vi "Interpolate String.vi"(6 "Gantry in":refnum<class "Gantry.lvclass">, 8 "error in (no error)":errorcluster, 10 "Input String":string, 11 "gScript Interpreter in":refnum<class "gScript Interpreter.lvclass">) -> (0 "error out":errorcluster, 2 "Output String":string, 3 "gScript Interpreter out":refnum<class "gScript Interpreter.lvclass">, 4 "Gantry out":refnum<class "Gantry.lvclass">)   [LabVIEW 2026, in "gScript Interpreter.lvclass"]
uses:
  gScript Interpreter.lvclass
  Shared Components/Gantry Class/Gantry.lvclass
  <vilib>/regexp/Match Regular Expression.xnode
  gScript Interpreter.lvclass/gScript Interpreter.ctl
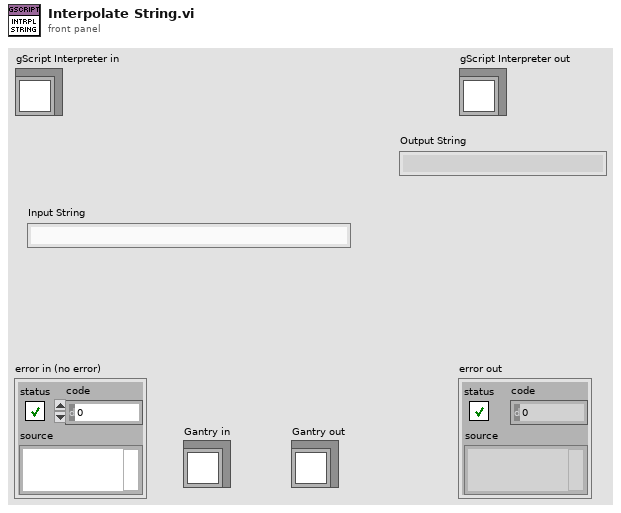
[diagram p1: front panel]
types:
  T1 = typedef "Memory Cell.ctl" = cluster{"type":T2, "x":dbl, "y":dbl, "z":dbl, "w":dbl}
  T2 = typedef "Memory Cell Type Enum.ctl" = enum16{"integer", "float", "vector", "rotation"}
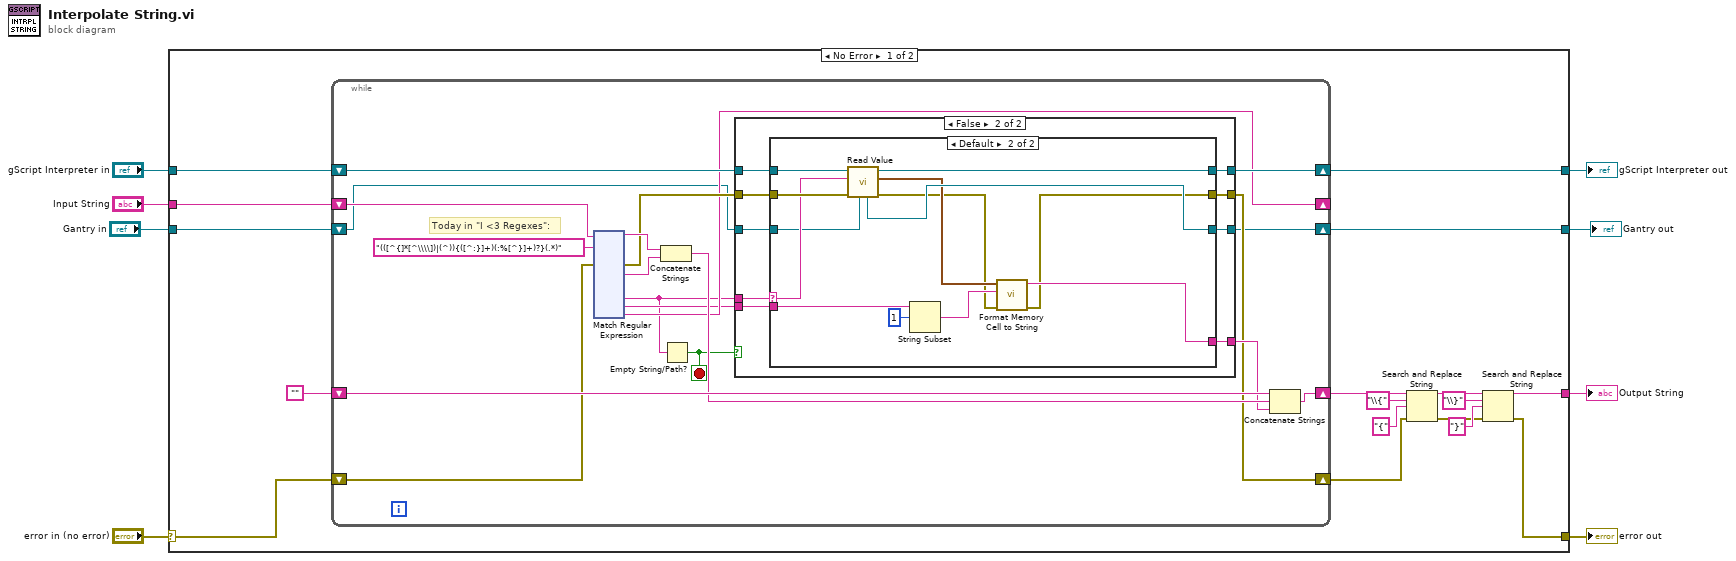
[diagram p0: block diagram]
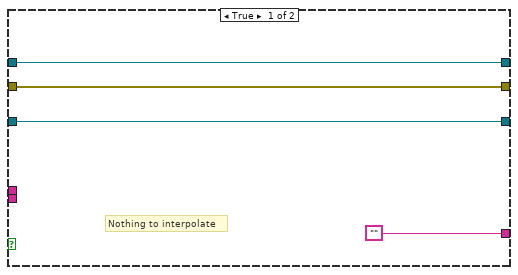
[diagram p2: hidden frame]
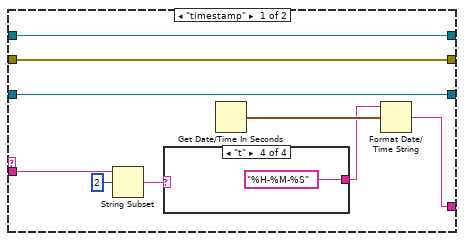
[diagram p3: hidden frame]
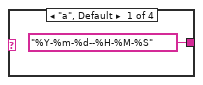
[diagram p4: hidden frame]
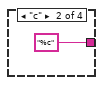
[diagram p5: hidden frame]
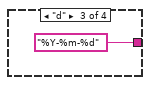
[diagram p6: hidden frame]
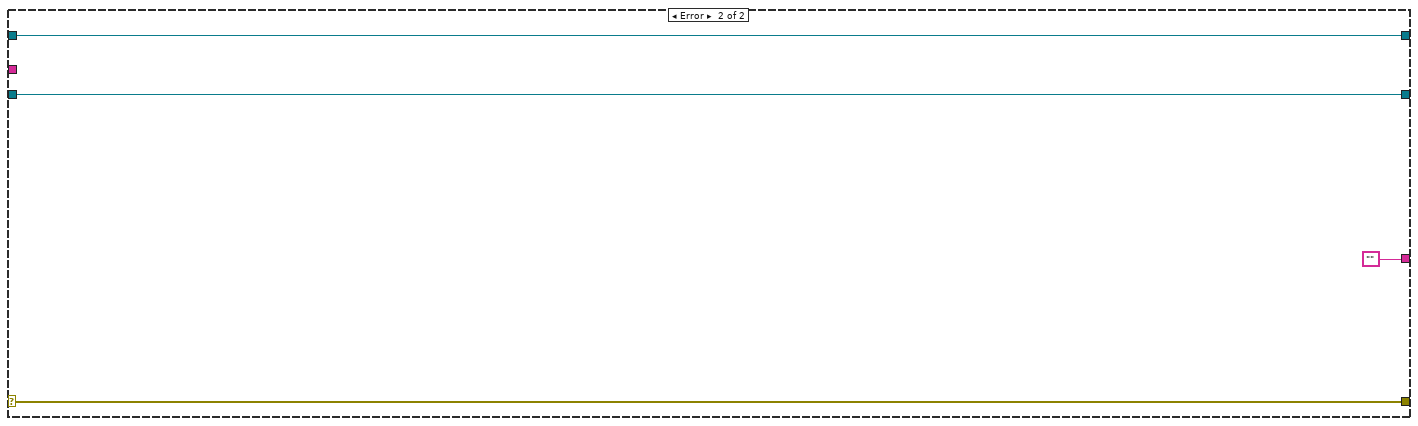
[diagram p7: hidden frame]
diagram:
  n1 = case shown="No Error" "error in (no error)" {
    selector: "error in (no error)" -> [w21 w211]
    tunnel: [w12 w211] -> w7
    tunnel: [w22 w210] -> w5
    tunnel: "gScript Interpreter in" -> [w23 w210]
    tunnel: "Input String" -> [w25 _]
    tunnel: [w11 ""] -> w3
    tunnel: "Gantry in" -> [w10 w208]
    tunnel: [w9 w208] -> w1
    frame No Error {
      n2 = while {
        shift-right: [w30] -> _
        shift-left: w25 -> [w44]
        shift-right: [w40] -> w20
        shift-left: "" -> [w39]
        shift-right: [w36] -> w22
        shift-left: w23 -> [w37]
        shift-right: [w31] -> w19
        shift-left: w21 -> [w35]
        shift-right: [w26] -> w9
        shift-left: w10 -> [w27]
        stop <- w33 stop-if-true
        # "Today in \"I <3 Regexes\":"
        n3 = xnode "Match Regular Expression"("input string"=w44, "regular expression"="(([^{]*[^\\\\])|(^)){([^:}]+)(:%[^}]+)?}(.*)", "error in"=w35) -> ("before match"=w42:string, "error out"=w34:errorcluster, "submatch 1"=w41:string, "submatch 4"=w28:string, "submatch 5"=w29:string, "submatch 6"=w30:string)  [unwired: 3 in, 5 out]
        n4 = Concatenate Strings(w42, w41) -> (w38:string)
        n5 = Empty String/Path?(string/path=w28) -> (empty?=w33:bool)
        n6 = case shown="False" w33 {
          tunnel: w37 -> [w48 w57]
          tunnel: [w48 w56] -> w36
          tunnel: w28 -> [_ w51]
          tunnel: w29 -> [_ w54]
          tunnel: w34 -> [w46 w55]
          tunnel: ["" w53] -> w32
          tunnel: [w46 w52] -> w31
          tunnel: w27 -> [w45 w50]
          tunnel: [w45 w49] -> w26
          frame True {
            # "Nothing to interpolate"
          }
          frame False {
            n7 = case shown="Default" w51 {
              selector: w51 -> [_ w80]
              tunnel: w57 -> [w66 w83]
              tunnel: [w66 w82] -> w56
              tunnel: w55 -> [w63 w81]
              tunnel: w54 -> [w61 w77]
              tunnel: [w62 w73] -> w53
              tunnel: [w63 w71] -> w52
              tunnel: w50 -> [w58 w79]
              tunnel: [w58 w78] -> w49
              frame "timestamp" {
                n8 = String Subset(string=w61, offset (0)=2) -> (substring=w60:string)  [unwired: 1 in]
                n9 = case shown="\"t\"" w60 {
                  tunnel: ["%Y-%m-%d--%H-%M-%S" "%c" "%Y-%m-%d" "%H-%M-%S"] -> w64
                  frame "a", Default {
                  }
                  frame "c" {
                  }
                  frame "d" {
                  }
                  frame "t" {
                  }
                }
                n10 = Get Date/Time In Seconds() -> (seconds since 1Jan1904=w65:timestamp)
                n11 = Format Date/Time String(time format string (%c)=w64, seconds (now)=w65) -> (date/time string=w62:string)  [unwired: 1 in]
              }
              frame Default {
                n12 = call-dynamic "Read Value.vi"("Gantry in"=w79, "error in (no error)"=w81, "String in"=w80, "gScript Interpreter in"=w83) -> ("error out"=w72:errorcluster, "Memory Cell"=w74:T1, "gScript Interpreter out"=w82:refnum<class "gScript Interpreter.lvclass">, "Gantry out"=w78:refnum<class "Gantry.lvclass">)  [unwired: 4 in]
                n13 = String Subset(string=w77, offset (0)=1) -> (substring=w75:string)  [unwired: 1 in]
                n14 = call "Format Memory Cell to String.vi"("error in (no error)"=w72, "Format String"=w75, "Memory Cell"=w74) -> ("error out"=w71:errorcluster, "output string"=w73:string)  [unwired: 7 in]
              }
            }
          }
        }
        n15 = Concatenate Strings(w39, w38, w32) -> (w40:string)
      }
      n16 = Search and Replace String(input string=w20, search string="\\{", replace string="{" ("replace string (\"\")"), error in=w19) -> (result string=w14:string, error out=w13:errorcluster)  [unwired: 4 in, 2 out]
      n17 = Search and Replace String(input string=w14, search string="\\}", replace string="}" ("replace string (\"\")"), error in=w13) -> (result string=w11:string, error out=w12:errorcluster)  [unwired: 4 in, 2 out]
    }
    frame Error {
    }
  }
  "error out" <- w7
  "gScript Interpreter out" <- w5
  "Output String" <- w3
  "Gantry out" <- w1
